vi "Excel Set Cell Alignment.vi"(0 "report in":refnum<class "NI_report.lvclass">, 1 "vertical alignment (top)":i32(ring) items=["top", "center", "bottom"], 2 "horizontal alignment (left)":i32(ring) items=["left", "center", "right"], 5 "wrap text? (F)":bool, 7 "start (-1, -1)":cluster{"row":i32, "column":i32}={"row"=-1, "column"=-1}, 9 "end (-1, -1)":cluster{"row":i32, "column":i32}={"row"=-1, "column"=-1}, 11 "error in (no error)":errorcluster, 12 "name (\"\")":string) -> (4 "report out":refnum<class "NI_report.lvclass">, 15 "error out":errorcluster)   [LabVIEW 2010, in "NI_Excel.lvclass"]
doc: "Sets the alignment of the cells specified by the <B>start</B> and <B>end</B> clusters or by a named range."
uses:
  <vilib>/Utility/NIReport.llb/Excel/NI_Excel.lvclass
  <vilib>/Utility/NIReport.llb/NI_report.lvclass
  <vilib>/Utility/NIReport.llb/Excel/NI_Excel.lvclass/NI_Excel.ctl
  NI_ReportGenerationToolkit.lvlib
  <vilib>/Utility/NIReport.llb/NI_ReportGenerationCore.lvlib
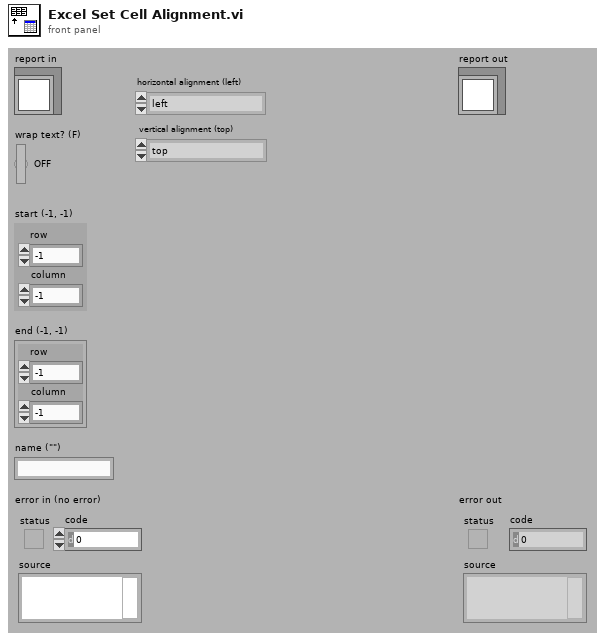
[diagram p1: front panel]
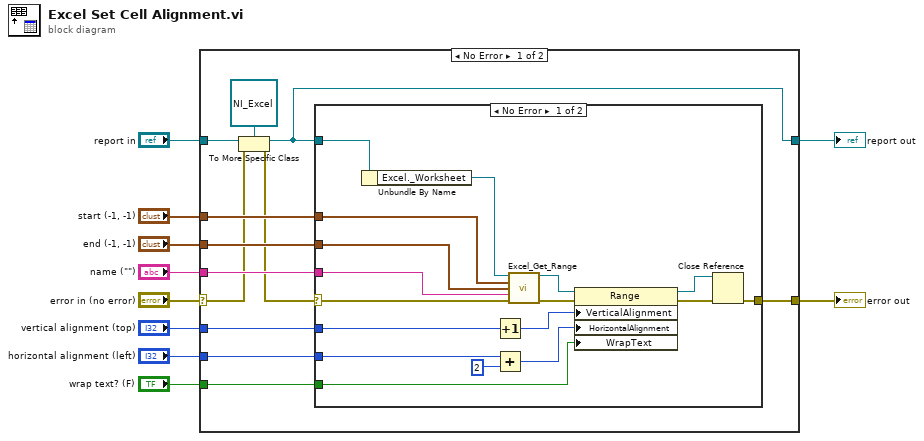
[diagram p0: block diagram]
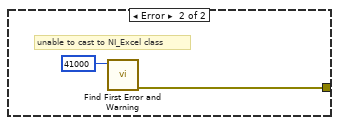
[diagram p2: hidden frame]
diagram:
  n1 = case shown="No Error" "error in (no error)" {
    selector: "error in (no error)" -> [w11 w43]
    tunnel: [w22 w43] -> w9
    tunnel: [w13 w42] -> w7
    tunnel: "report in" -> [w14 w42]
    tunnel: "start (-1, -1)" -> [w21 _]
    tunnel: "end (-1, -1)" -> [w20 _]
    tunnel: "name (\"\")" -> [w19 _]
    tunnel: "vertical alignment (top)" -> [w18 _]
    tunnel: "horizontal alignment (left)" -> [w17 _]
    tunnel: "wrap text? (F)" -> [w16 _]
    frame No Error {
      n2 = To More Specific Class(target class=refnum<class "NI_Excel.lvclass"> refnum ("report in"), reference=w14, error in=w11) -> (specific class reference=w13:refnum<class "NI_Excel.lvclass">, error out=w12:errorcluster)
      n3 = case shown="No Error" w12 {
        selector: w12 -> [w23 _]
        tunnel: [w32 w40] -> w22
        tunnel: w21 -> [w31 _]
        tunnel: w20 -> [w30 _]
        tunnel: w19 -> [w29 _]
        tunnel: w18 -> [w28 _]
        tunnel: w17 -> [w27 _]
        tunnel: w16 -> [w26 _]
        tunnel: w13 -> [w24 _]
        frame No Error {
          n4 = Unbundle By Name(w24) -> ("Excel._Worksheet"=w36:refnum<k7>)
          n5 = Increment(x=w28) -> (x+1=w35:i32)
          n6 = Add(x=w27, y=2) -> (x+y=w25:i32)
          n7 = call <vilib>:"Excel_Get_Range.vi"("Excel._Worksheet"=w36, "start"=w31, "end"=w30, "name"=w29, "error in (no error)"=w23) -> ("Range"=w37:refnum<k7>, "error out"=w39:errorcluster)  [unwired: 5 in, 4 out]
          n8 = property class="Range"(reference=w37, error in=w39, "VerticalAlignment"=w35, "HorizontalAlignment"=w25, "WrapText"=w26) -> (reference out=w34:refnum<k7>, error out=w33:errorcluster)
          n9 = Close Reference(reference=w34, error in (no error)=w33) -> (error out=w32:errorcluster)
        }
        frame Error {
          # "unable to cast to NI_Excel class"
          n10 = call <vilib>:"Find First Error and Warning.vi"("error code"=41000) -> ("error out"=w40:errorcluster)  [unwired: 2 in, 4 out]
        }
      }
    }
    frame Error {
    }
  }
  "error out" <- w9
  "report out" <- w7
